vi "R1DataCollection.vi"(8 "error constant":errorcluster, 10 "Write Once":bool, 11 "LabVIEW Web Service":refnum<class "Web Service.lvclass">) -> (0 "error out":errorcluster)   [LabVIEW 2016]
uses:
  <vilib>/wsapi/Web Service.lvclass
  <vilib>/Platform/TimedLoop/XDataNode/timing_clust.ctl
  <vilib>/Platform/TimedLoop/XDataNode/nitl_modes.ctl
  <vilib>/Platform/TimedLoop/XDataNode/wakeup.ctl
  Controls/pH_Manual Standard.ctl
  <vilib>/Platform/TimedLoop/XDataNode/XDataNode.xnode
  <vilib>/Platform/TimedLoop/XDataNode/XDNodeRunTimeDep.lvlib
  <vilib>/ptbypt/NI_PtbyPt.lvlib
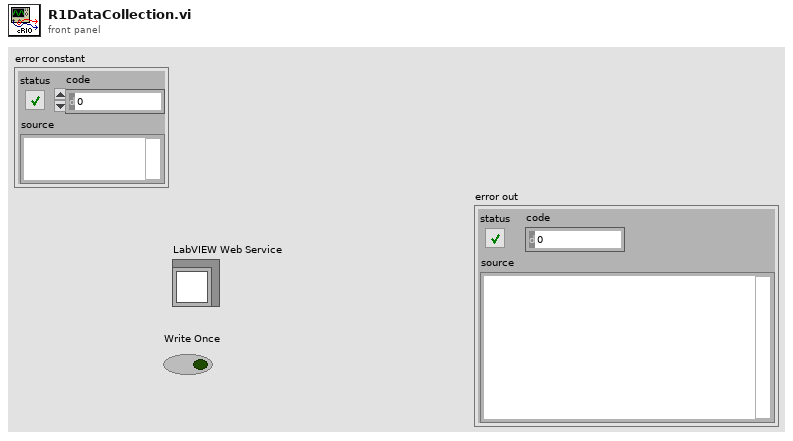
[diagram p1: front panel]
types:
  T1 = typedef "XDNodeRunTimeDep.lvlib/timing_clust.ctl" = cluster{"Expected End [f-1]":u64, "Actual End [f-1]":u64, "Finished Late? [f-1]":bool, "Expected End [i-1]":u64, "Actual End [i-1]":u64, "Finished Late? [i-1]":bool, "Expected Start [i]":u64, "Actual Start [i]":u64, "Expected Start [f]":u64, "Actual Start [f]":u64, "Source Name":string, "Structure Name":string, "Period":i64, "Deadline":i64, "Offset":i64, "Start":i64, "Priority":i32, "Timeout":i32, "Mode":T2, "Wakeup Reason":T3, "Error":errorcluster, "Source Type":string, "Secondary Source Type":string, "Global End Time":u64, "Global Start Time":u64, "Frame Duration":u64, "Iteration Duration":u64, "Assigned CPU":i32, "I/O Scan Engine Mode":u32}
  T2 = typedef "XDNodeRunTimeDep.lvlib/nitl_modes.ctl" = enum32{"No Change", "Process missed periods, maintain original phase", "Discard missed periods, maintain original phase", "Process missed periods, ignore original phase", "Discard missed periods, ignore original phase"}
  T3 = typedef "XDNodeRunTimeDep.lvlib/wakeup.ctl" = enum32{"Normal", "Aborted", "Asynchronous wakeup", "Timing source error", "Timed loop error", "Timeout"}
  T4 = cluster{"Media Pump":bool, "Water Pump":bool, "Effluent Pump":bool, "Release Valve":bool, "Gas Pump":bool}
  T5 = typedef "pH_Manual Standard.ctl" = cluster{"Acid Pump":bool, "Base Pump":bool}
  T6 = cluster{"Array of Double[0]":dbl, "Array of Double[1]":dbl, "Array of Double[2]":dbl, "Array of Double[3]":dbl, "Array of Double[4]":dbl, "Array of Double[5]":dbl, "Array of Double[6]":dbl, "Array of Double[7]":dbl, "Array of Double[8]":dbl}
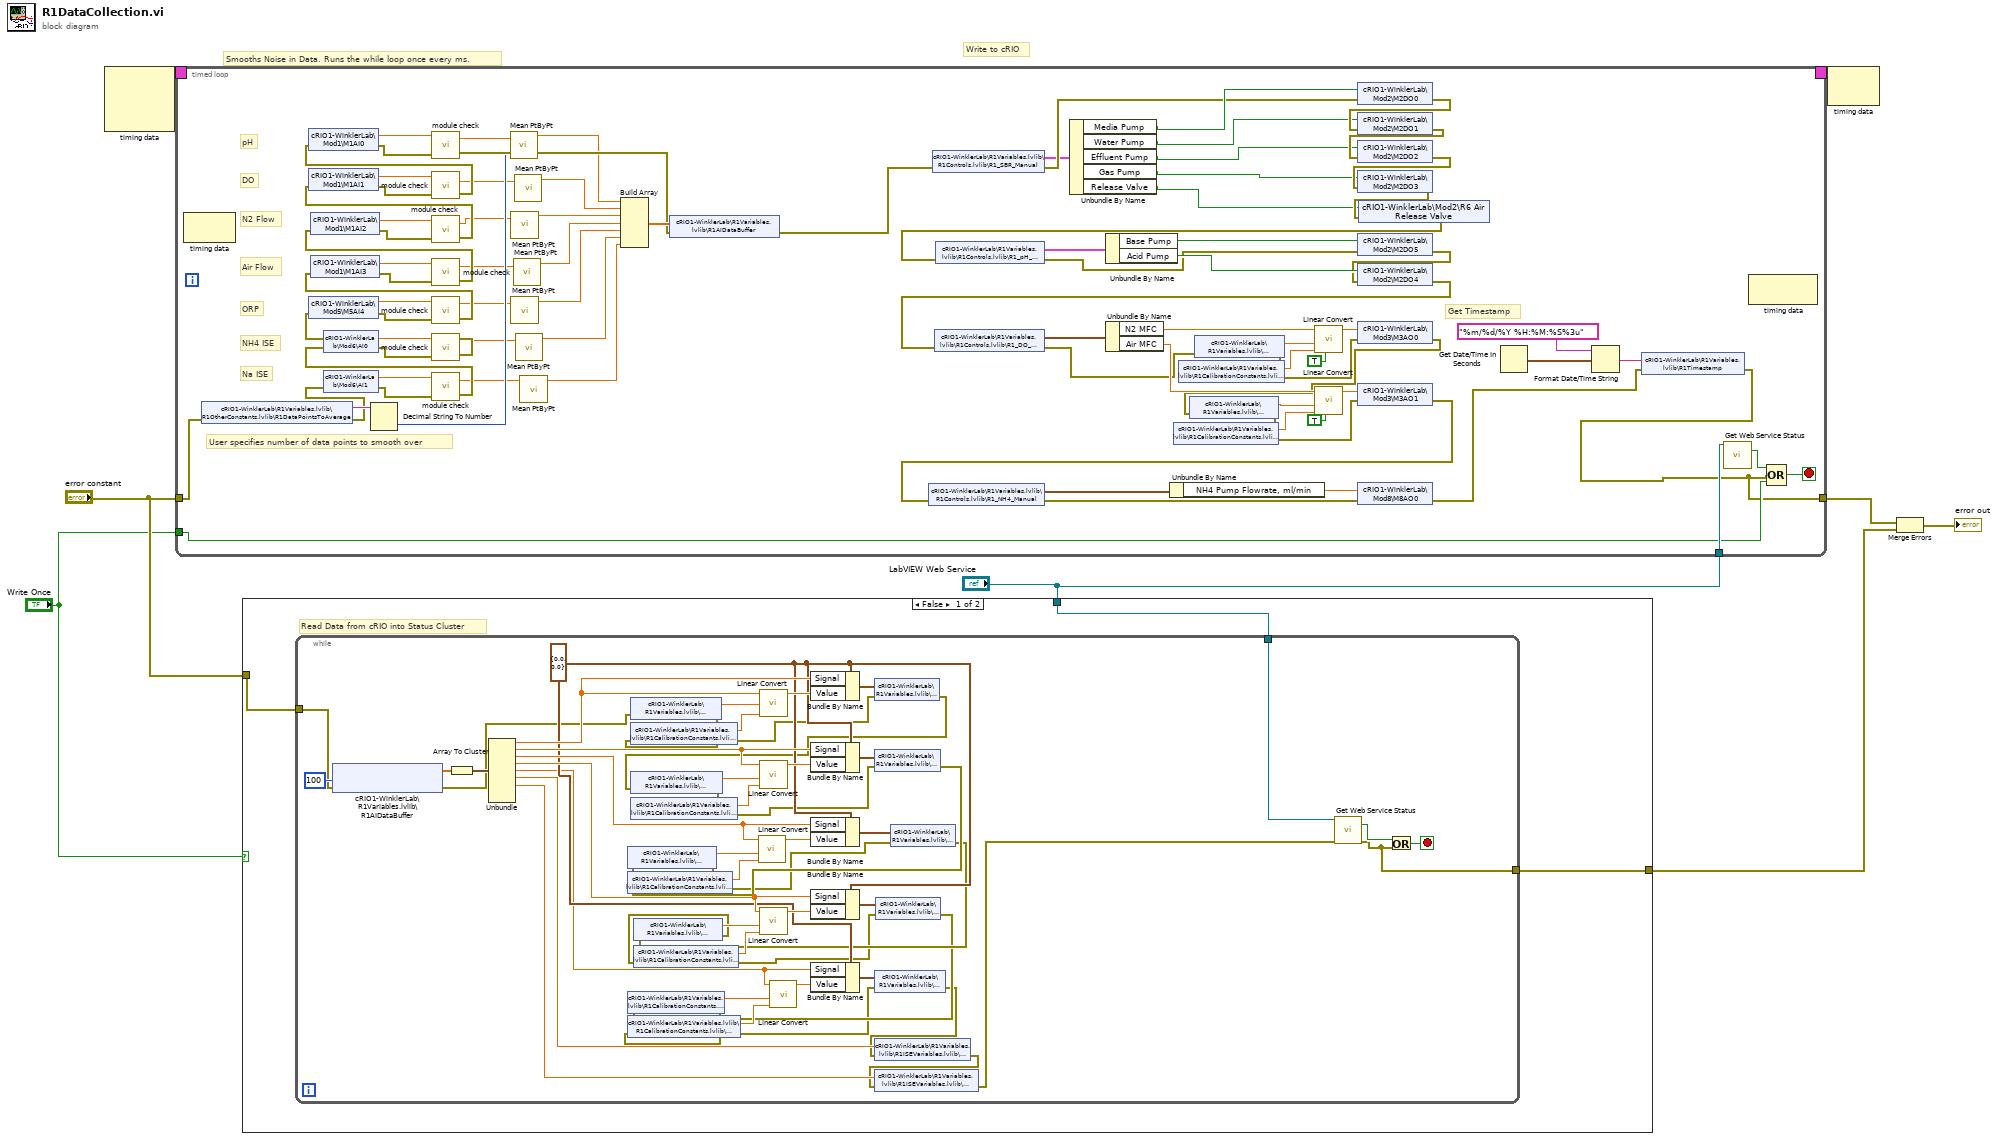
[diagram p0: block diagram]
diagram:
  # "Write to cRIO"
  # "Smooths Noise in Data. Runs the while loop once every ms."
  n1 = node-c288() -> (w8:T1)  [unwired: 3 in]
  n2 = timed-loop {
    timing: w8 -> [_]
    timing-out: [_] -> w7
    tunnel: "error constant" -> [w92]
    tunnel: "LabVIEW Web Service" -> [w90]
    tunnel: "Write Once" -> [w88]
    tunnel: [w87] -> w3
    stop <- w86 stop-if-true
    # "NH4 ISE"
    # "Na ISE"
    # "ORP"
    # "Get Timestamp"
    # "User specifies number of data points to smooth over"
    # "Air Flow"
    # "N2 Flow"
    # "DO"
    # "pH"
    n3 = node-c288() -> ()  [unwired: 1 in, 1 out]
    n4 = shared-variable "cRIO1-WinklerLab\\R1Variables.lvlib\\R1OtherConstants.lvlib\\R1DataPointsToAverage"(error in=w92) -> (w93:string, error out=w81:errorcluster)
    n5 = shared-variable "cRIO1-WinklerLab\\Mod6\\AI1"(error in=w81) -> (w85:dbl, error out=w84:errorcluster)
    n6 = Decimal String To Number(string=w93) -> (number=w63:i32)  [unwired: 2 in, 1 out]
    n7 = call "module check.vi"("error in"=w84, "Value"=w85) -> ("error constant"=w82:errorcluster, "Value out"=w60:dbl)  [unwired: 1 in]
    n8 = shared-variable "cRIO1-WinklerLab\\Mod6\\AI0"(error in=w82) -> (w83:dbl, error out=w80:errorcluster)
    n9 = call "module check.vi"("error in"=w80, "Value"=w83) -> ("error constant"=w79:errorcluster, "Value out"=w58:dbl)  [unwired: 1 in]
    n10 = shared-variable "cRIO1-WinklerLab\\Mod5\\M5AI4"(error in=w79) -> (w78:dbl, error out=w77:errorcluster)
    n11 = call "module check.vi"("error in"=w77, "Value"=w78) -> ("error constant"=w76:errorcluster, "Value out"=w56:dbl)  [unwired: 1 in]
    n12 = shared-variable "cRIO1-WinklerLab\\Mod1\\M1AI3"(error in=w76) -> (w75:dbl, error out=w74:errorcluster)
    n13 = call "module check.vi"("error in"=w74, "Value"=w75) -> ("error constant"=w73:errorcluster, "Value out"=w53:dbl)  [unwired: 1 in]
    n14 = shared-variable "cRIO1-WinklerLab\\Mod1\\M1AI2"(error in=w73) -> (w72:dbl, error out=w71:errorcluster)
    n15 = call "module check.vi"("error in"=w71, "Value"=w72) -> ("error constant"=w70:errorcluster, "Value out"=w52:dbl)  [unwired: 1 in]
    n16 = shared-variable "cRIO1-WinklerLab\\Mod1\\M1AI1"(error in=w70) -> (w68:dbl, error out=w69:errorcluster)
    n17 = call "module check.vi"("error in"=w69, "Value"=w68) -> ("error constant"=w66:errorcluster, "Value out"=w49:dbl)  [unwired: 1 in]
    n18 = shared-variable "cRIO1-WinklerLab\\Mod1\\M1AI0"(error in=w66) -> (w67:dbl, error out=w65:errorcluster)
    n19 = call "module check.vi"("error in"=w65, "Value"=w67) -> ("error constant"=w64:errorcluster, "Value out"=w62:dbl)  [unwired: 1 in]
    n20 = call <vilib>:"Mean PtByPt.vi"("x"=w62, "sample length"=w63) -> ("mean"=w61:dbl)  [unwired: 2 in, 1 out]
    n21 = call <vilib>:"Mean PtByPt.vi"("x"=w52) -> ("mean"=w51:dbl)  [unwired: 3 in, 1 out]
    n22 = call <vilib>:"Mean PtByPt.vi"("x"=w56) -> ("mean"=w55:dbl)  [unwired: 3 in, 1 out]
    n23 = call <vilib>:"Mean PtByPt.vi"("x"=w53) -> ("mean"=w54:dbl)  [unwired: 3 in, 1 out]
    n24 = call <vilib>:"Mean PtByPt.vi"("x"=w49) -> ("mean"=w50:dbl)  [unwired: 3 in, 1 out]
    n25 = call <vilib>:"Mean PtByPt.vi"("x"=w58) -> ("mean"=w57:dbl)  [unwired: 3 in, 1 out]
    n26 = call <vilib>:"Mean PtByPt.vi"("x"=w60) -> ("mean"=w59:dbl)  [unwired: 3 in, 1 out]
    n27 = Build Array(w61, w50, w51, w54, w55, w57, w59) -> (w97:dbl[])
    n28 = shared-variable "cRIO1-WinklerLab\\R1Variables.lvlib\\R1AIDataBuffer"(w97, error in=w64) -> (error out=w20:errorcluster)
    n29 = shared-variable "cRIO1-WinklerLab\\R1Variables.lvlib\\R1Controls.lvlib\\R1_SBR_Manual"(error in=w20) -> (w18:T4, error out=w19:errorcluster)
    n30 = Unbundle By Name(w18) -> ("Media Pump"=w25:bool, "Water Pump"=w24:bool, "Effluent Pump"=w23:bool, "Gas Pump"=w22:bool, "Release Valve"=w21:bool)
    n31 = shared-variable "cRIO1-WinklerLab\\Mod2\\M2DO0"(w25, error in=w19) -> (error out=w46:errorcluster)
    n32 = shared-variable "cRIO1-WinklerLab\\Mod2\\M2DO1"(w24, error in=w46) -> (error out=w47:errorcluster)
    n33 = shared-variable "cRIO1-WinklerLab\\Mod2\\M2DO2"(w23, error in=w47) -> (error out=w48:errorcluster)
    n34 = shared-variable "cRIO1-WinklerLab\\Mod2\\M2DO3"(w22, error in=w48) -> (error out=w26:errorcluster)
    n35 = shared-variable "cRIO1-WinklerLab\\Mod2\\R6 Air Release Valve"(w21, error in=w26) -> (error out=w17:errorcluster)
    n36 = shared-variable "cRIO1-WinklerLab\\R1Variables.lvlib\\R1Controls.lvlib\\R1_pH_Manual"(error in=w17) -> (w15:T5, error out=w16:errorcluster)
    n37 = Unbundle By Name(w15) -> ("Base Pump"=w44:bool, "Acid Pump"=w45:bool)
    n38 = shared-variable "cRIO1-WinklerLab\\Mod2\\M2DO5"(w44, error in=w16) -> (error out=w43:errorcluster)
    n39 = shared-variable "cRIO1-WinklerLab\\Mod2\\M2DO4"(w45, error in=w43) -> (error out=w14:errorcluster)
    n40 = shared-variable "cRIO1-WinklerLab\\R1Variables.lvlib\\R1Controls.lvlib\\R1_DO_Manual"(error in=w14) -> (w12:cluster{"Air MFC":dbl, "N2 MFC":dbl}, error out=w13:errorcluster)
    n41 = Unbundle By Name(w12) -> ("N2 MFC"=w41:dbl, "Air MFC"=w40:dbl)
    n42 = shared-variable "cRIO1-WinklerLab\\R1Variables.lvlib\\R1CalibrationConstants.lvlib\\R1N2Slope"(error in=w13) -> (w35:dbl, error out=w32:errorcluster)
    n43 = shared-variable "cRIO1-WinklerLab\\R1Variables.lvlib\\R1CalibrationConstants.lvlib\\R1N2Intercept"(error in=w32) -> (w34:dbl, error out=w31:errorcluster)
    n44 = call "Linear Convert.vi"("Inverse?"=TRUE, "Intercept"=w34, "Slope"=w35, "Signal"=w41) -> ("Result"=w33:dbl)  [unwired: 7 in]
    n45 = shared-variable "cRIO1-WinklerLab\\Mod3\\M3AO0"(w33, error in=w31) -> (error out=w30:errorcluster)
    n46 = shared-variable "cRIO1-WinklerLab\\R1Variables.lvlib\\R1CalibrationConstants.lvlib\\R1AirSlope"(error in=w30) -> (w37:dbl, error out=w29:errorcluster)
    n47 = shared-variable "cRIO1-WinklerLab\\R1Variables.lvlib\\R1CalibrationConstants.lvlib\\R1AirIntercept"(error in=w29) -> (w36:dbl, error out=w28:errorcluster)
    n48 = call "Linear Convert.vi"("Inverse?"=TRUE, "Intercept"=w36, "Slope"=w37, "Signal"=w40) -> ("Result"=w42:dbl)  [unwired: 7 in]
    n49 = shared-variable "cRIO1-WinklerLab\\Mod3\\M3AO1"(w42, error in=w28) -> (error out=w10:errorcluster)
    n50 = shared-variable "cRIO1-WinklerLab\\R1Variables.lvlib\\R1Controls.lvlib\\R1_NH4_Manual"(error in=w10) -> (w9:cluster{"NH4 Pump Flowrate, ml/min":dbl}, error out=w11:errorcluster)
    n51 = Unbundle By Name(w9) -> ("NH4 Pump Flowrate, ml/min"=w27:dbl)
    n52 = shared-variable "cRIO1-WinklerLab\\Mod8\\M8AO0"(w27, error in=w11) -> (error out=w91:errorcluster)
    n53 = Get Date/Time In Seconds() -> (seconds since 1Jan1904=w95:timestamp)
    n54 = Format Date/Time String(time format string (%c)="%m/%d/%Y %H:%M:%S%3u", seconds (now)=w95) -> (date/time string=w94:string)  [unwired: 1 in]
    n55 = shared-variable "cRIO1-WinklerLab\\R1Variables.lvlib\\R1Timestamp"(w94, error in=w91) -> (error out=w87:errorcluster)
    n56 = call <vilib>:"Get Web Service Status.vi"("LabVIEW Web Service"=w90) -> ("service stopping?"=w89:bool)  [unwired: 12 in, 2 out]
    n57 = node-c288() -> ()  [unwired: 1 in, 1 out]
    n58 = Compound Arithmetic op=OR(w89, w87, w88) -> (w86:bool)
  }
  n59 = case shown="False" "Write Once" {
    tunnel: "error constant" -> [w102 w157]
    tunnel: "LabVIEW Web Service" -> [w101 _]
    tunnel: [w100 w157] -> w2
    frame False {
      # "Read Data from cRIO into Status Cluster"
      n60 = while {
        tunnel: w102 -> [w106]
        tunnel: [w104] -> w100
        tunnel: w101 -> [w103]
        stop <- w146 stop-if-true
        w133 = cluster{"Signal":dbl, "Value":dbl} {"Signal"=0.0, "Value"=0.0} ("Analog Input")
        n61 = shared-variable "cRIO1-WinklerLab\\R1Variables.lvlib\\R1AIDataBuffer"(error in=w106, u32 100 ("milliseconds to wait")) -> (w154:dbl[], error out=w123:errorcluster)  [unwired: 1 out]
        n62 = Array To Cluster(array=w154) -> (cluster=w156:T6)
        n63 = Unbundle(w156) -> ("Array of Double[0]"=w152:dbl, "Array of Double[1]"=w150:dbl, "Array of Double[2]"=w139:dbl, "Array of Double[3]"=w138:dbl, "Array of Double[4]"=w130:dbl, "Array of Double[5]"=w137:dbl, "Array of Double[6]"=w136:dbl)  [unwired: 2 out]
        n64 = shared-variable "cRIO1-WinklerLab\\R1Variables.lvlib\\R1CalibrationConstants.lvlib\\R1pHSlope"(error in=w123) -> (w144:dbl, error out=w122:errorcluster)
        n65 = shared-variable "cRIO1-WinklerLab\\R1Variables.lvlib\\R1CalibrationConstants.lvlib\\R1pHIntercept"(error in=w122) -> (w145:dbl, error out=w121:errorcluster)
        n66 = call "Linear Convert.vi"("Intercept"=w145, "Slope"=w144, "Signal"=w152) -> ("Result"=w153:dbl)  [unwired: 8 in]
        n67 = Bundle By Name(cluster=w133, "Signal"=w152, "Value"=w153) -> (w151:cluster{"Signal":dbl, "Value":dbl})
        n68 = shared-variable "cRIO1-WinklerLab\\R1Variables.lvlib\\R1Signals.lvlib\\R1pH"(w151, error in=w121) -> (error out=w120:errorcluster)
        n69 = shared-variable "cRIO1-WinklerLab\\R1Variables.lvlib\\R1CalibrationConstants.lvlib\\R1DOSlope"(error in=w120) -> (w143:dbl, error out=w119:errorcluster)
        n70 = shared-variable "cRIO1-WinklerLab\\R1Variables.lvlib\\R1CalibrationConstants.lvlib\\R1DOIntercept"(error in=w119) -> (w142:dbl, error out=w118:errorcluster)
        n71 = call "Linear Convert.vi"("Intercept"=w142, "Slope"=w143, "Signal"=w150) -> ("Result"=w148:dbl)  [unwired: 8 in]
        n72 = Bundle By Name(cluster=w133, "Signal"=w150, "Value"=w148) -> (w149:cluster{"Signal":dbl, "Value":dbl})
        n73 = shared-variable "cRIO1-WinklerLab\\R1Variables.lvlib\\R1Signals.lvlib\\R1DO"(w149, error in=w118) -> (error out=w117:errorcluster)
        n74 = shared-variable "cRIO1-WinklerLab\\R1Variables.lvlib\\R1CalibrationConstants.lvlib\\R1N2Slope"(error in=w117) -> (w127:dbl, error out=w116:errorcluster)
        n75 = shared-variable "cRIO1-WinklerLab\\R1Variables.lvlib\\R1CalibrationConstants.lvlib\\R1N2Intercept"(error in=w116) -> (w126:dbl, error out=w115:errorcluster)
        n76 = call "Linear Convert.vi"("Intercept"=w126, "Slope"=w127, "Signal"=w139) -> ("Result"=w140:dbl)  [unwired: 8 in]
        n77 = Bundle By Name(cluster=w133, "Signal"=w139, "Value"=w140) -> (w124:cluster{"Signal":dbl, "Value":dbl})
        n78 = shared-variable "cRIO1-WinklerLab\\R1Variables.lvlib\\R1Signals.lvlib\\R1N2"(w124, error in=w115) -> (error out=w114:errorcluster)
        n79 = shared-variable "cRIO1-WinklerLab\\R1Variables.lvlib\\R1CalibrationConstants.lvlib\\R1AirSlope"(error in=w114) -> (w129:dbl, error out=w113:errorcluster)
        n80 = shared-variable "cRIO1-WinklerLab\\R1Variables.lvlib\\R1CalibrationConstants.lvlib\\R1AirIntercept"(error in=w113) -> (w128:dbl, error out=w112:errorcluster)
        n81 = call "Linear Convert.vi"("Intercept"=w128, "Slope"=w129, "Signal"=w138) -> ("Result"=w141:dbl)  [unwired: 8 in]
        n82 = Bundle By Name(cluster=w133, "Signal"=w138, "Value"=w141) -> (w125:cluster{"Signal":dbl, "Value":dbl})
        n83 = shared-variable "cRIO1-WinklerLab\\R1Variables.lvlib\\R1Signals.lvlib\\R1Air"(w125, error in=w112) -> (error out=w111:errorcluster)
        n84 = shared-variable "cRIO1-WinklerLab\\R1Variables.lvlib\\R1CalibrationConstants.lvlib\\R1ORPSlope"(error in=w111) -> (w132:dbl, error out=w110:errorcluster)
        n85 = shared-variable "cRIO1-WinklerLab\\R1Variables.lvlib\\R1CalibrationConstants.lvlib\\R1ORPIntercept"(error in=w110) -> (w131:dbl, error out=w109:errorcluster)
        n86 = call "Linear Convert.vi"("Intercept"=w131, "Slope"=w132, "Signal"=w130) -> ("Result"=w135:dbl)  [unwired: 8 in]
        n87 = Bundle By Name(cluster=w133, "Signal"=w130, "Value"=w135) -> (w134:cluster{"Signal":dbl, "Value":dbl})
        n88 = shared-variable "cRIO1-WinklerLab\\R1Variables.lvlib\\R1Signals.lvlib\\R1ORP"(w134, error in=w109) -> (error out=w108:errorcluster)
        n89 = shared-variable "cRIO1-WinklerLab\\R1Variables.lvlib\\R1ISEVariables.lvlib\\R1NaISERaw"(w137, error in=w108) -> (error out=w107:errorcluster)
        n90 = shared-variable "cRIO1-WinklerLab\\R1Variables.lvlib\\R1ISEVariables.lvlib\\R1NH4ISERaw"(w136, error in=w107) -> (error out=w105:errorcluster)
        n91 = call <vilib>:"Get Web Service Status.vi"("LabVIEW Web Service"=w103, "error in (no error)"=w105) -> ("service stopping?"=w147:bool, "error out"=w104:errorcluster)  [unwired: 11 in, 1 out]
        n92 = Or(x=w147, y=w104) -> (x .or. y?=w146:bool)
      }
    }
    frame True {
    }
  }
  n93 = node-c288(w7) -> ()  [unwired: 1 out]
  n94 = Merge Errors(w3, w2) -> (→"error out":errorcluster)
